vi "convert 2d num.vi"(1 "Mouse Position":cluster{"X":i32, "Y":i32}) -> (0 "Array Position":cluster{"Row":i32, "Column":i32})   [LabVIEW 2009]
panel:
  in  "Input Position Name":cluster{"Row":i32, "Column":i32}
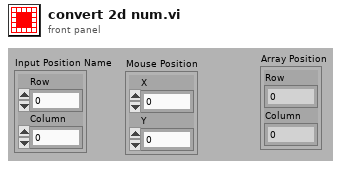
[diagram p1: front panel]
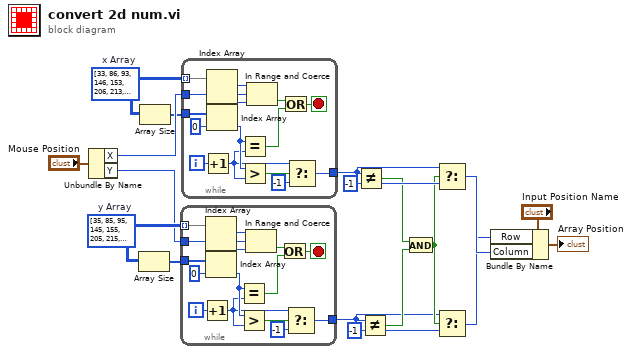
[diagram p0: block diagram]
diagram:
  w10 = -1 ("y")
  w11 = -1 ("y")
  w13 = i32[][] [[35, 85], [95, 145], [155, 205], [215, 265], [275, 325], [335, 385], [395, 445], [455, 505], [515, 565], [575, 625], [-1000, 1000]]  # y Array
  w16 = i32[][] [[33, 86], [93, 146], [153, 206], [213, 266], [273, 326], [333, 386], [393, 446], [453, 506], [513, 566], [-1000, 1000]]  # x Array
  n1 = Unbundle By Name("Mouse Position") -> ("X"=w17:i32, "Y"=w12:i32)
  n2 = Array Size(array=w13) -> (size(s)=w14:i32[])
  n3 = Array Size(array=w16) -> (size(s)=w15:i32[])
  n4 = while {
    tunnel: w12 -> [w33]
    tunnel: w13 -> [w32] mode=indexing
    tunnel: w14 -> [w31]
    tunnel: [w21] -> w5
    i -> [w23]
    stop <- w28 stop-if-true
    n5 = Increment(x=w23) -> (x+1=w25:i32)
    n6 = Index Array(array=w32) -> (element #1=w20:i32, element #2=w19:i32)  [unwired: 2 in]
    n7 = Index Array(array=w31, index=0 ("Index")) -> (element=w26:i32)
    n8 = Equal?(x=w26, y=w25) -> (x = y?=w27:bool)
    n9 = Greater?(x=w26, y=w25) -> (0:w24:bool)
    n10 = In Range and Coerce(upper limit=w19, x=w33, lower limit=w20) -> (In Range?=w29:bool)  [unwired: 1 out]
    n11 = Or(x=w29, y=w27) -> (x .or. y?=w28:bool)
    n12 = Select(t=w23, s=w24, f=-1) -> (s? t:f=w21:i32)
  }
  n13 = while {
    tunnel: w17 -> [w48]
    tunnel: w16 -> [w47] mode=indexing
    tunnel: w15 -> [w46]
    tunnel: [w36] -> w6
    i -> [w38]
    stop <- w43 stop-if-true
    n14 = Increment(x=w38) -> (x+1=w40:i32)
    n15 = Index Array(array=w47) -> (element #1=w35:i32, element #2=w34:i32)  [unwired: 2 in]
    n16 = Index Array(array=w46, index=0 ("Index")) -> (element=w41:i32)
    n17 = Equal?(x=w41, y=w40) -> (x = y?=w42:bool)
    n18 = Greater?(x=w41, y=w40) -> (0:w39:bool)
    n19 = In Range and Coerce(upper limit=w34, x=w48, lower limit=w35) -> (In Range?=w44:bool)  [unwired: 1 out]
    n20 = Or(x=w44, y=w42) -> (x .or. y?=w43:bool)
    n21 = Select(t=w38, s=w39, f=-1) -> (s? t:f=w36:i32)
  }
  n22 = Not Equal?(x=w6, y=w11) -> (x != y?=w9:bool)
  n23 = Not Equal?(x=w5, y=w10) -> (x != y?=w8:bool)
  n24 = And(x=w9, y=w8) -> (x .and. y?=w7:bool)
  n25 = Select(t=w6, s=w7, f=w11) -> (s? t:f=w3:i32)
  n26 = Select(t=w5, s=w7, f=w10) -> (s? t:f=w2:i32)
  n27 = Bundle By Name(cluster="Input Position Name", "Row"=w2, "Column"=w3) -> (→"Array Position":cluster{"Row":i32, "Column":i32})
